vi "setAndorErrorCodes.vi"(8 "error in (no error)":errorcluster, 10 "Andor Error Codes":dbl[](array[numeric]), 11 "AndorIKonTempController.lvclass in":refnum<class "AndorIKonTempController.lvclass">) -> (0 "error out":errorcluster, 3 "AndorIKonTempController.lvclass out":refnum<class "AndorIKonTempController.lvclass">)   [LabVIEW 2011, in "Hardware.lvlib" / "Channels.lvlib" / "AndorIKonTempController.lvclass"]
uses:
  AndorIKonTempController.lvclass
  AndorIKonTempController.lvclass/AndorIKonTempController.ctl
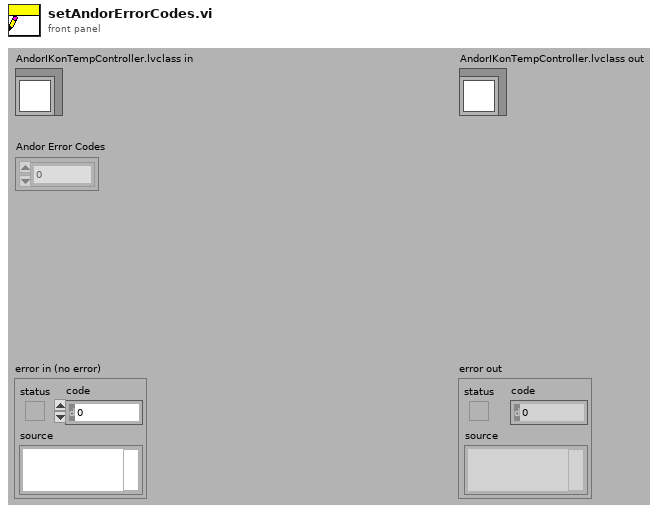
[diagram p1: front panel]
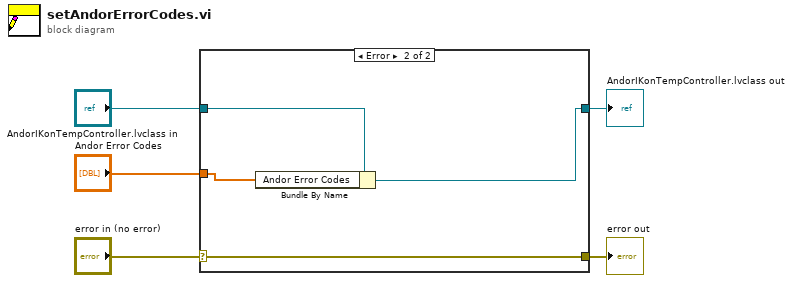
[diagram p0: block diagram]
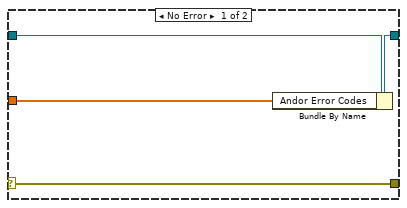
[diagram p2: hidden frame]
diagram:
  n1 = case shown="Error" "error in (no error)" {
    selector: "error in (no error)" -> [w9 w13]
    tunnel: [w9 w13] -> w4
    tunnel: [w7 w11] -> w2
    tunnel: "AndorIKonTempController.lvclass in" -> [w8 w12]
    tunnel: "Andor Error Codes" -> [w6 w10]
    frame No Error {
      n2 = Bundle By Name(cluster=w8, "Andor Error Codes"=w6) -> (w7:refnum<class "AndorIKonTempController.lvclass">)
    }
    frame Error {
      n3 = Bundle By Name(cluster=w12, "Andor Error Codes"=w10) -> (w11:refnum<class "AndorIKonTempController.lvclass">)
    }
  }
  "error out" <- w4
  "AndorIKonTempController.lvclass out" <- w2
